vi "vms_getEvent_SettingVersions.vi"(8 "error in (no error)":errorcluster, 11 "logevent_SettingVersions_Ctl":T1) -> (0 "error out":errorcluster, 2 "function return":i32, 3 "logevent_SettingVersions_Ctl out":T1)   [LabVIEW 2016, in "SALLV_vms.lvlib"]
doc: "int vms_shm_getEvent_SettingVersionsLV(vms_logevent_SettingVersionsLV *logevent_SettingVersions_Ctl );"
uses:
  SALLV_vms.lvlib
  DataTypes/logevent_SettingVersions.ctl
  SALLV_vms.so
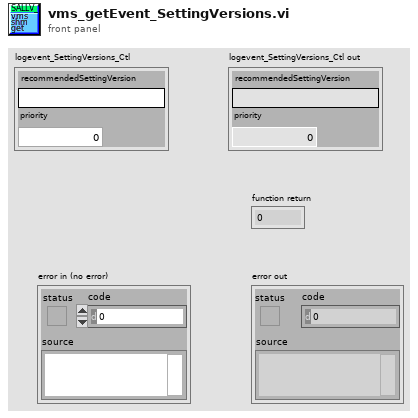
[diagram p1: front panel]
types:
  T1 = typedef "SALLV_vms.lvlib/logevent_SettingVersions.ctl" = cluster{"recommendedSettingVersion":string, "priority":i32}
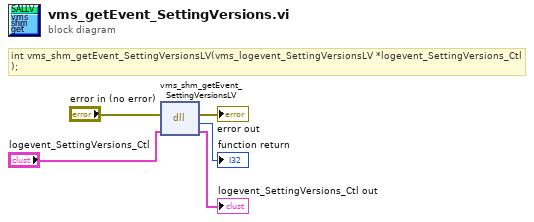
[diagram p0: block diagram]
diagram:
  # "int vms_shm_getEvent_SettingVersionsLV(vms_logevent_SettingVersionsLV *logevent_SettingVersions_Ctl );"
  n1 = dll-call lib="opt/CODE/SALLV_vms/SALLV_vms.*" fn="vms_shm_getEvent_SettingVersionsLV"(error in="error in (no error)", "logevent_SettingVersions_Ctl"="logevent_SettingVersions_Ctl") -> (error out=→"error out":errorcluster, →"function return":i32, "logevent_SettingVersions_Ctl"=→"logevent_SettingVersions_Ctl out":T1)  [unwired: 2 in, 1 out]
